vi "Fetch (Calculation).vi"(8 "error in (no error)":errorcluster, 11 "VISA resource name":refnum<visa-resource-name>) -> (0 "error out":errorcluster, 1 "Minimum":dbl format="%#.10g", 2 "Standard Deviation":dbl format="%#.10g", 3 "VISA resource name out":refnum<visa-resource-name>, 4 "Maximum":dbl format="%#.10g", 5 "Mean":dbl format="%#.10g")   [LabVIEW 2020, in "Counter.lvlib" / "PICOTEST U62XXA series.lvlib"]
doc: "Queries and Returns Statistical data for the specified number of measurements.\n\n<B>Note:</B>\n\nIf no valid result exists, Not a Number 9.91E37 is returned."
uses:
  PICOTEST U62XXA series.lvlib
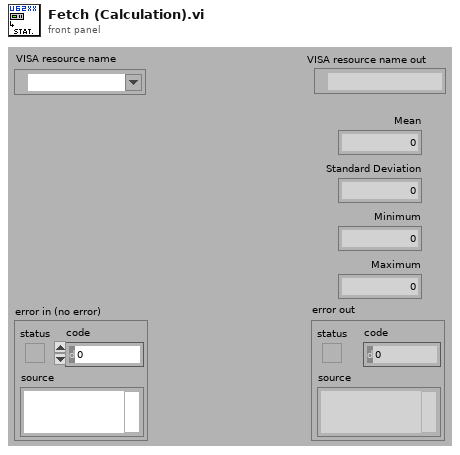
[diagram p1: front panel]
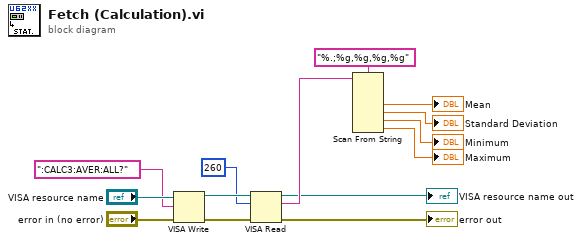
[diagram p0: block diagram]
diagram:
  n1 = VISA Write(VISA resource name="VISA resource name", write buffer=":CALC3:AVER:ALL?", error in (no error)="error in (no error)") -> (VISA resource name out=w9:refnum<visa-resource-name>, error out=w10:errorcluster)  [unwired: 1 out]
  n2 = VISA Read(VISA resource name=w9, byte count=u32 260, error in (no error)=w10) -> (VISA resource name out=→"VISA resource name out":refnum<visa-resource-name>, read buffer=w11:string, error out=→"error out":errorcluster)  [unwired: 1 out]
  n3 = Scan From String(format string="%.;%g,%g,%g,%g", input string=w11) -> (output 1=→"Mean":dbl, output 2=→"Standard Deviation":dbl, output 3=→"Minimum":dbl, output 4=→"Maximum":dbl)  [unwired: 6 in, 3 out]
